vi "Adjust Trace.vi"(8 "error in (no error)":errorcluster, 11 "Historical Data In":T1) -> (0 "error out":errorcluster, 3 "Historical Data Out":T1)   [LabVIEW 2024]
doc: "Adjusts a trace to display the trace."
uses:
  Controls/Client/Historical Data.ctl
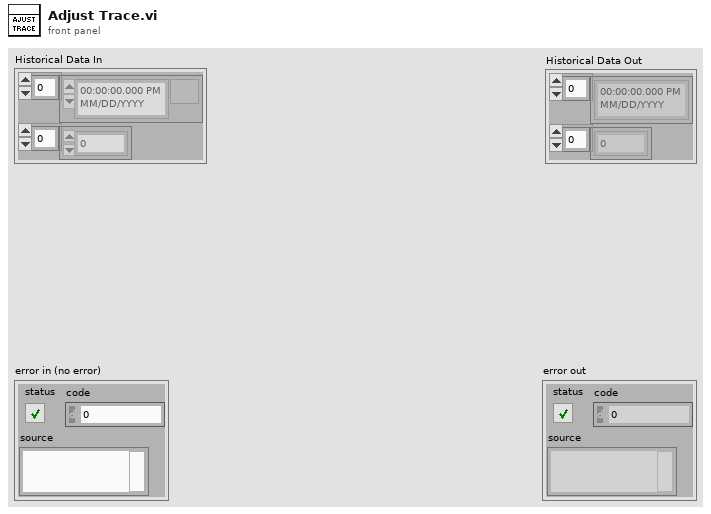
[diagram p1: front panel]
types:
  T1 = typedef "Historical Data.ctl" = cluster{"timestamps":timestamp[], "data":dbl[]}
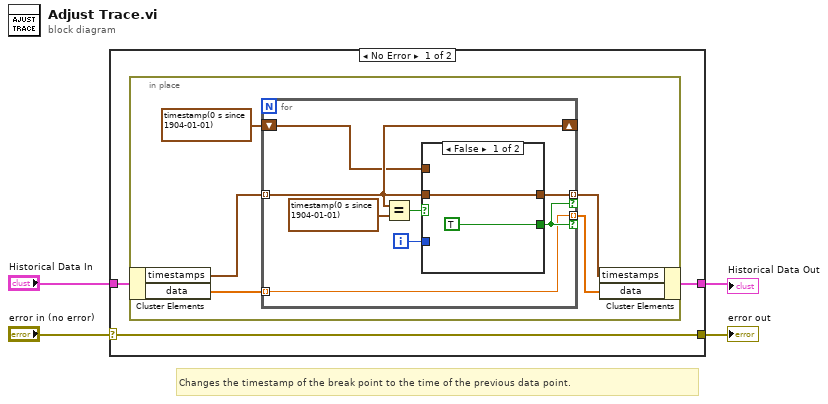
[diagram p0: block diagram]
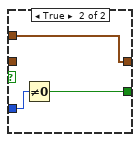
[diagram p2: hidden frame]
diagram:
  # "Changes the timestamp of the break point to the time of the previous data point."
  n1 = case shown="No Error" "error in (no error)" {
    selector: "error in (no error)" -> [w5 w27]
    tunnel: [w5 w27] -> w3
    tunnel: [w6 w26] -> w2
    tunnel: "Historical Data In" -> [w7 w26]
    frame No Error {
      n2 = in-place {
        n3 = in-place-cluster #1(w7) -> ("timestamps"=w10:timestamp[], "data"=w11:dbl[])
        n4 = for {
          tunnel: w10 -> [w18] mode=indexing
          shift-right: [w18] -> _
          shift-left: timestamp(0 s since 1904-01-01) ("y") -> [w16]
          tunnel: [w17] -> w9 mode=indexing if=w15
          tunnel: [w14] -> w8 mode=indexing if=w15
          tunnel: w11 -> [w14] mode=indexing
          i -> [w19]
          n5 = Equal?(x=w18, y=timestamp(0 s since 1904-01-01)) -> (x = y?=w13:bool)
          n6 = case shown="False" w13 {
            tunnel: w18 -> [w22 _]
            tunnel: w19 -> [_ w24]
            tunnel: [w22 w25] -> w17
            tunnel: w16 -> [_ w25]
            tunnel: [TRUE w23] -> w15
            frame False {
            }
            frame True {
              n7 = Not Equal To 0?(x=w24) -> (x != 0?=w23:bool)
            }
          }
        }
        n8 = in-place-cluster #1("timestamps"=w9, "data"=w8) -> (w6:T1)
      }
    }
    frame Error {
    }
  }
  "error out" <- w3
  "Historical Data Out" <- w2
